vi "Add Device by Resource.vi"(8 "error in (no error)":errorcluster, 10 "Resource":refnum<class "DeployResource.lvclass">, 11 "DeviceManager in":refnum<class "DeviceManager.lvclass">) -> (0 "error out":errorcluster, 2 "Device":refnum<class "Device.lvclass">, 3 "DeviceManager out":refnum<class "DeviceManager.lvclass">)   [LabVIEW 2020, in "PicoG-Core.lvlib" / "DeviceManager.lvclass"]
uses:
  DeviceManager.lvclass
  DeployResource/DeployResource.lvclass
  Device/Device.lvclass
  DeviceManager.lvclass/DeviceManager.ctl
  DeployPlatform/DeployPlatform.lvclass
  PlatformPluginManager/PlatformPluginManager.lvclass
  PicoG-Core.lvlib
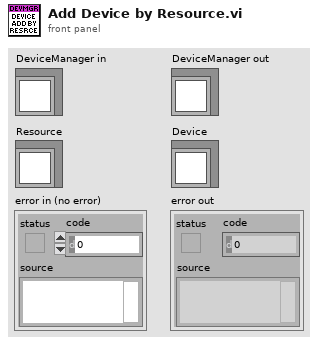
[diagram p1: front panel]
types:
  T1 = map{refnum<class "DeployResource.lvclass">, refnum<class "Device.lvclass">}
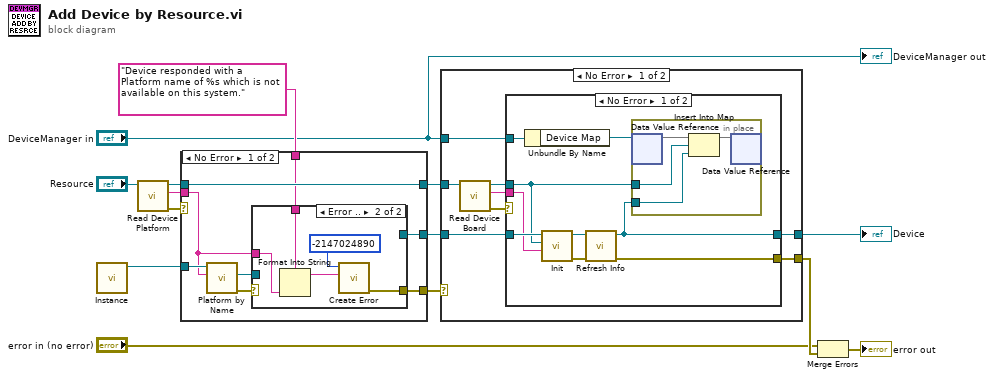
[diagram p0: block diagram]
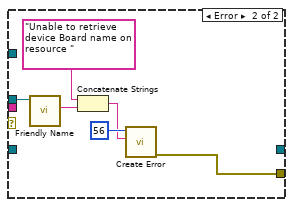
[diagram p4: hidden frame]
diagram:
  n1 = call "Instance.vi"() -> ("Platform Manager"=w13:refnum<class "PlatformPluginManager.lvclass">)  [unwired: 10 in, 1 out]
  n2 = call "Read Device Platform.vi"("Resource in"="Resource") -> ("error out"=w14:errorcluster, "Platform"=w11:string, "Resource out"=w10:refnum<class "DeployResource.lvclass">)  [unwired: 8 in]
  n3 = case shown="No Error" w14 {
    selector: w14 -> [_ w30]
    tunnel: w13 -> [w21 _]
    tunnel: w11 -> [w15 _]
    tunnel: [w17 _] -> w8
    tunnel: [w22 w30] -> w9
    tunnel: w10 -> [w20 _]
    tunnel: [w20 _] -> w7
    tunnel: "Device responded with a Platform name of %s which is not available on this system." -> [w16 _]
    frame No Error {
      n4 = call "Platform by Name.vi"("Platform"=w15, "TargetPluginManager in"=w21) -> ("error out"=w19:errorcluster, "Platform"=w18:refnum<class "DeployPlatform.lvclass">)  [unwired: 7 in, 1 out]
      n5 = case shown="Error .." w19 {
        selector: w19 -> [w23 _]
        tunnel: w18 -> [w24 _]
        tunnel: [w24 _] -> w17
        tunnel: [w23 w29] -> w22
        tunnel: w16 -> [_ w27]
        tunnel: w15 -> [_ w26]
        frame No Error {
        }
        frame Error {
          n6 = Format Into String(format string=w27, w26) -> (resulting string=w25:string)  [unwired: 2 in, 1 out]
          n7 = call "Create Error.vi"("Message (\"\")"=w25, "Code"=-2147024890) -> ("error out"=w29:errorcluster)  [unwired: 9 in]
        }
      }
    }
    frame Error {
    }
  }
  n8 = case shown="No Error" w9 {
    selector: w9 -> [_ w58]
    tunnel: w8 -> [w34 _]
    tunnel: w7 -> [w38 _]
    tunnel: [w33 w58] -> w3
    tunnel: "DeviceManager in" -> [w32 _]
    tunnel: [w31 _] -> w5
    frame No Error {
      n9 = call "Read Device Board.vi"("Resource in"=w38) -> ("error out"=w37:errorcluster, "Board"=w35:string, "Resource out"=w36:refnum<class "DeployResource.lvclass">)  [unwired: 8 in]
      n10 = case shown="No Error" w37 {
        tunnel: w35 -> [w46 _]
        tunnel: w36 -> [w43 w56]
        tunnel: w34 -> [w47 _]
        tunnel: [w40 w52] -> w33
        tunnel: w32 -> [w45 _]
        tunnel: [w39 _] -> w31
        frame No Error {
          n11 = Unbundle By Name(w45) -> ("Device Map"=w44:refnum<data-value>)
          n12 = call "Init.vi"("Board (Default)"=w46, "Resource (None)"=w43, "Platform (None)"=w47) -> ("error out"=w41:errorcluster, "Device out"=w42:refnum<class "Device.lvclass">)  [unwired: 7 in]
          n13 = call "Refresh Info.vi"("error in (no error)"=w41, "Device in"=w42) -> ("error out"=w40:errorcluster, "Device out"=w39:refnum<class "Device.lvclass">)  [unwired: 8 in]
          n14 = in-place {
            in-place-border: w39 -> [w49]
            in-place-border: w43 -> [w50]
            n15 = in-place-dvr #1(w44) -> (w51:T1)  [unwired: 1 out]
            n16 = Insert Into Map(map in=w51, key=w50, value=w49) -> (map out=w48:T1)  [unwired: 2 out]
            n17 = in-place-dvr #1(w48) -> ()  [unwired: 2 out]
          }
        }
        frame Error {
          n18 = call-dynamic "Friendly Name.vi"("DeployResource in"=w56) -> ("Friendly Name"=w55:string)  [unwired: 8 in, 2 out]
          n19 = Concatenate Strings("Unable to retrieve device Board name on resource " ("Message (\"\")"), w55) -> (w53:string)
          n20 = call "Create Error.vi"("Message (\"\")"=w53, "Code"=56) -> ("error out"=w52:errorcluster)  [unwired: 9 in]
        }
      }
    }
    frame Error {
    }
  }
  "Device" <- w5
  n21 = Merge Errors("error in (no error)", w3) -> (→"error out":errorcluster)
  "DeviceManager out" <- "DeviceManager in"
